vi "Teleop.vi"(10 "Match Info":T1={"Autonomous Elapsed Seconds"=0.0, "TeleOp Elapsed Seconds"=0.0, "Disabled Elapsed Seconds"=0.0, "Visited Autonomous"=FALSE, "Visited TeleOp"=FALSE, "Visited Disabled"=FALSE, "Autonomous Settings"={"Autonomous Style"=enum."Independent", "VI Refnum"=refnum}}, 11 "Call Context":T2) -> ()   [LabVIEW 2018]
doc: "This VI is called for each TeleOp packet received from the DS where the robot is not disabled. It is often used to read from the joysticks and update I/O or to update setpoints for timed control loops. It should complete and return within 20 milliseconds or it may miss DS packets."
uses:
  <vilib>/Rock Robotics/WPI/DriverStation/WPI_DriverStationDerivedRobotMode.ctl
  <vilib>/Rock Robotics/WPI/DriverStation/WPI_DriverStationMatch Info.ctl
  <vilib>/Rock Robotics/WPI/Utilities/WPI_GetSetVariantRefNum.vi
  <vilib>/Rock Robotics/Network Tables/NT Write Boolean Array.vi
  <vilib>/Rock Robotics/Network Tables/NT Write Numeric Array.vi
  <vilib>/Rock Robotics/Network Tables/NT Read Boolean.vi
  <vilib>/Rock Robotics/Network Tables/NT Read Number.vi
panel:
  out "Sample Slider 0":dbl(slide) scale=0.0..5.0
  out "Sample Boolean 1":bool
  out "Sample Boolean 0":bool
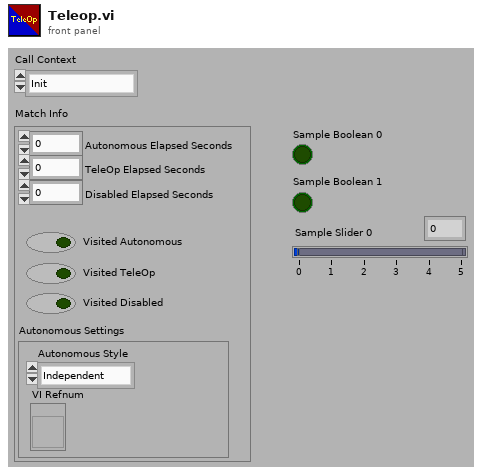
[diagram p1: front panel]
types:
  T1 = typedef "WPI_DriverStationMatch Info.ctl" = cluster{"Autonomous Elapsed Seconds":dbl, "TeleOp Elapsed Seconds":dbl, "Disabled Elapsed Seconds":dbl, "Visited Autonomous":bool, "Visited TeleOp":bool, "Visited Disabled":bool, "Autonomous Settings":cluster{"Autonomous Style":enum16{"Iterative", "Independent"}, "VI Refnum":refnum<vi>}}
  T2 = typedef "WPI_DriverStationDerivedRobotMode.ctl" = enum16{"Init", "Execute", "Stop"}
  T3 = typedef "WPI_RobotDriveDevRef.ctl" = cluster{"DevStatus":errorcluster, "Motors[]":T4[], "Square Inputs":bool, "Max Output":dbl}
  T4 = typedef "WPI_MotorControlDeviceRef.ctl" = cluster{"DeviceStatus":errorcluster, "Type":T5, "PWM":cluster{"PWM Channel":T6, "DeadBand":T7}, "CAN":cluster{"Device Number":u8, "SetOutput VI Ref":variant, "GetOutput VI Ref":variant, "Enable VI Ref":variant, "Disable VI Ref":variant, "Data":variant}, "Invert":bool, "DIO PWM":cluster{"PWM \"Enable\" Channel":T6, "DIOChannel":T8, "PWM Rate":dbl}}
  T5 = typedef "WPI_MotorControlType.ctl" = enum16{"PWM", "CAN", "DIO PWM"}
  T6 = typedef "FPGA_DIOPWMChannel.ctl" = enum8{"PWM 0", "PWM 1", "PWM 2", "PWM 3", "PWM 4", "PWM 5", "PWM 6", "PWM 7", "PWM 8", "PWM 9", "PWM MXP 0", "PWM MXP 1", "PWM MXP 2", "PWM MXP 3", "PWM MXP 4", "PWM MXP 5", "PWM MXP 6", "PWM MXP 7", "PWM MXP 8", "PWM MXP 9", "Invalid"}
  T7 = typedef "WPI_PWMDeadband.ctl" = cluster{"Name":string, "maxPositivePwm":i32, "minPositivePwm":i32, "centerPwm":i32, "maxNegativePwm":i32, "minNegativePwm":i32, "angularRange":u16}
  T8 = typedef "FPGA_DIOChannel.ctl" = enum8{"DIO 0", "DIO 1", "DIO 2", "DIO 3", "DIO 4", "DIO 5", "DIO 6", "DIO 7", "DIO 8", "DIO 9", "DIO MXP 0", "DIO MXP 1", "DIO MXP 2", "DIO MXP 3", "DIO MXP 4", "DIO MXP 5", "DIO MXP 6", "DIO MXP 7", "DIO MXP 8", "DIO MXP 9", "DIO MXP 10", "DIO MXP 11", "DIO MXP 12", "DIO MXP 13", "DIO MXP 14", "DIO MXP 15", "SPI Port CS1", "SPI Port CS2", "SPI Port CS3", "SPI Port MISO", "SPI Port MOSI", "Invalid"}
  T9 = typedef "WPI_JoystickDevRef.ctl" = cluster{"Device":T10}
  T10 = typedef "WPI_JoystickDeviceEnum.ctl" = enum16{"USB 0", "USB 1", "USB 2", "USB 3", "USB 4", "USB 5"}
  T11 = typedef "WPI_SwitchDevRef.ctl" = cluster{"DevStatus":errorcluster, "DIO Channel":T8, "CntIndex":T12, "Normally Closed":bool}
  T12 = typedef "FPGA_CounterCtrSystemIndex.ctl" = enum8{"Ctr 0", "Ctr 1", "Ctr 2", "Ctr 3", "Ctr 4", "Ctr 5", "Ctr 6", "Ctr 7", "Invalid"}
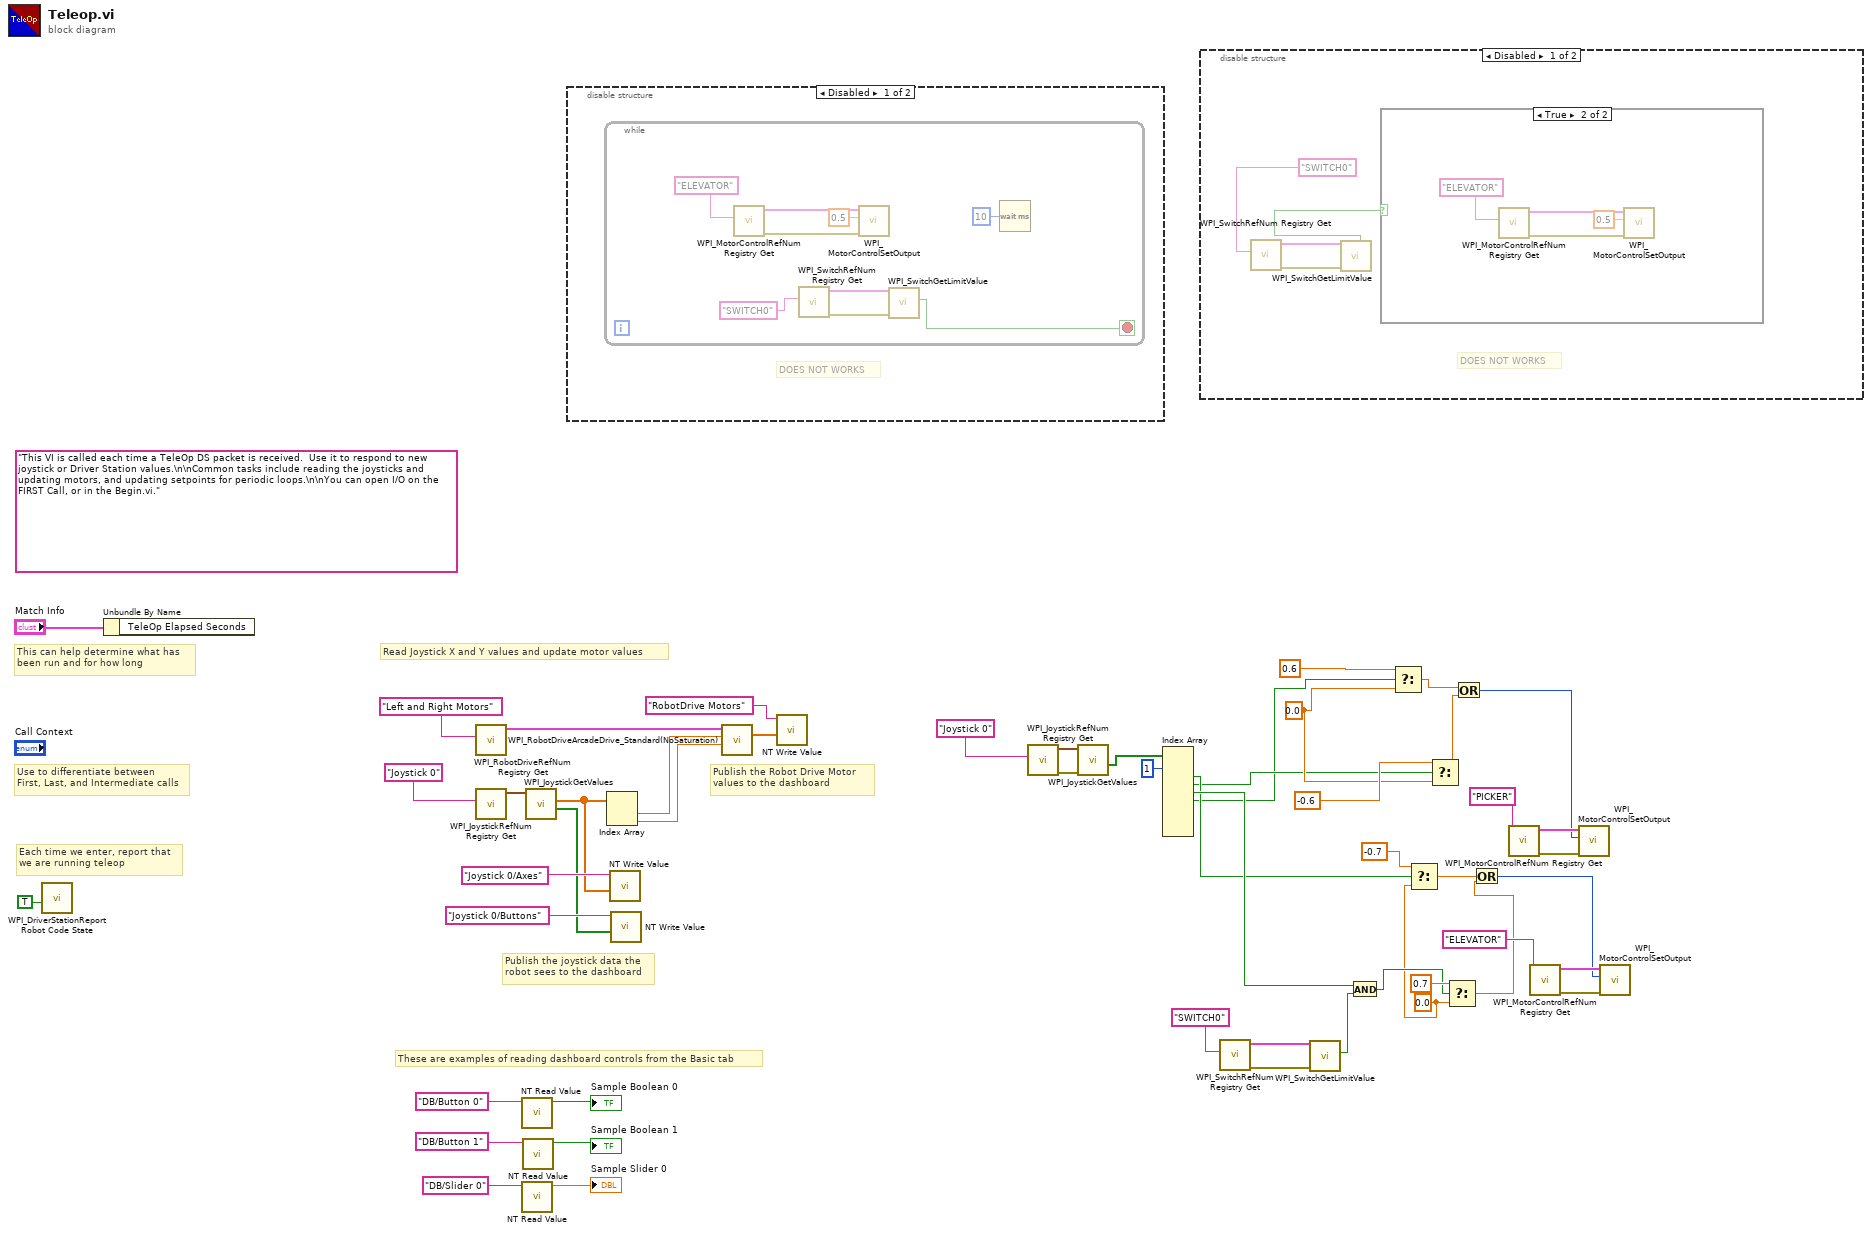
[diagram p0: block diagram]
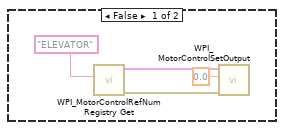
[diagram p2: hidden frame]
diagram:
  w4 = 0.0 ("f")
  w11 = 0.0 ("t")
  (unwired) "This VI is called each time a TeleOp DS packet is received.  Use it to respond to new joystick or Driver Station values.\n\nCommon tasks include reading the joysticks and updating motors, and updating setpoints for periodic loops.\n\nYou can open I/O on the FIRST Call, or in the Begin.vi."
  # "These are examples of reading dashboard controls from the Basic tab"
  # "Publish the Robot Drive Motor\nvalues to the dashboard"
  # "Publish the joystick data the\nrobot sees to the dashboard"
  # "Each time we enter, report that\nwe are running teleop"
  # "Use to differentiate between\nFirst, Last, and Intermediate calls"
  # "This can help determine what has\nbeen run and for how long"
  # "Read Joystick X and Y values and update motor values"
  n1 = call <vilib>:"WPI_DriverStationReport Robot Code State.vi"("TeleOp"=TRUE ("Autonomous")) -> ()  [unwired: 10 in, 1 out]
  n2 = Unbundle By Name("Match Info") -> ()  [unwired: 1 out]
  n3 = call <vilib>:"WPI_RobotDriveRefNum Registry Get.vi"("refnum name"="Left and Right Motors") -> ("RobotDriveDevRef"=w50:T3)  [unwired: 1 in, 9 out]
  n4 = call <vilib>:"WPI_JoystickRefNum Registry Get.vi"("refnum name"="Joystick 0") -> ("JoystickDevRef"=w47:T9)  [unwired: 1 in, 9 out]
  n5 = call-poly <vilib>:"NT Read Value.vi"("Name"="DB/Button 0" ("refnum name")) -> ("Boolean"=→"Sample Boolean 0":bool)  [unwired: 9 in, 1 out]
  n6 = call-poly <vilib>:"NT Read Value.vi"("Name"="DB/Slider 0" ("refnum name")) -> ("Numeric"=→"Sample Slider 0":dbl)  [unwired: 9 in, 1 out]
  n7 = call-poly <vilib>:"NT Read Value.vi"("Name"="DB/Button 1" ("refnum name")) -> ("Boolean"=→"Sample Boolean 1":bool)  [unwired: 9 in, 1 out]
  n8 = call <vilib>:"WPI_JoystickGetValues.vi"("JoystickDevRef"=w47) -> ("Buttons"=w41:bool[], "Axes"=w42:dbl[])  [unwired: 6 in, 3 out]
  n9 = disable-structure shown="Disabled" {
    frame Disabled {
      # "DOES NOT WORKS"
      n10 = while {
        stop <- w53 stop-if-true
        n11 = call <vilib>:"WPI_MotorControlRefNum Registry Get.vi"("refnum name"="ELEVATOR") -> ("error out"=w58:errorcluster, "MotorControlDevRef"=w57:T4)  [unwired: 9 in]
        n12 = call <vilib>:"WPI_SwitchRefNum Registry Get.vi"("refnum name"="SWITCH0") -> ("error out"=w61:errorcluster, "SwitchDevRef"=w60:T11)  [unwired: 9 in]
        n13 = call <vilib>:"WPI_MotorControlSetOutput.vi"("error in (no error)"=w58, "Output"=0.5, "MotorControlDevRef"=w57) -> ()  [unwired: 6 in, 3 out]
        n14 = call <vilib>:"WPI_SwitchGetLimitValue.vi"("error in (no error)"=w61, "SwitchDevRef"=w60) -> ("Switch Pressed"=w53:bool)  [unwired: 7 in, 2 out]
        n15 = Wait (ms)(milliseconds to wait=u32 10) -> ()  [unwired: 1 out]
      }
    }
    frame Enabled {
    }
  }
  n16 = Index Array(array=w42) -> (element #1=w49:dbl, element #2=w45:dbl)  [unwired: 2 in]
  n17 = call-poly <vilib>:"NT Write Value.vi"("Numeric Array"=w42, "Name"="Joystick 0/Axes") -> ()  [unwired: 9 in, 1 out]
  n18 = call-poly <vilib>:"NT Write Value.vi"("Boolean Array"=w41, "Name"="Joystick 0/Buttons") -> ()  [unwired: 9 in, 1 out]
  n19 = call <vilib>:"WPI_RobotDriveArcadeDrive_Standard(NoSaturation).vi"("Y axis value"=w45, "X axis value"=w49, "RobotDriveDevRef"=w50) -> ("Motor Values"=w34:dbl[])  [unwired: 1 in, 7 out]
  n20 = call-poly <vilib>:"NT Write Value.vi"("Numeric Array"=w34, "Name"="RobotDrive Motors") -> ()  [unwired: 9 in, 1 out]
  n21 = call <vilib>:"WPI_JoystickRefNum Registry Get.vi"("refnum name"="Joystick 0") -> ("error out"=w28:errorcluster, "JoystickDevRef"=w31:T9)  [unwired: 1 in, 8 out]
  n22 = call <vilib>:"WPI_JoystickGetValues.vi"("error in (no error)"=w28, "JoystickDevRef"=w31) -> ("Buttons"=w30:bool[])  [unwired: 5 in, 4 out]
  n23 = Index Array(array=w30, index #1=1 ("index")) -> (element #2=w3:bool, element #3=w2:bool, element #4=w9:bool, element #5=w1:bool)  [unwired: 8 in, 5 out]
  n24 = disable-structure shown="Disabled" {
    frame Disabled {
      # "DOES NOT WORKS"
      n25 = call <vilib>:"WPI_SwitchRefNum Registry Get.vi"("refnum name"="SWITCH0") -> ("error out"=w65:errorcluster, "SwitchDevRef"=w64:T11)  [unwired: 9 in]
      n26 = call <vilib>:"WPI_SwitchGetLimitValue.vi"("error in (no error)"=w65, "SwitchDevRef"=w64) -> ("Switch Pressed"=w62:bool)  [unwired: 7 in, 2 out]
      n27 = case shown="True" w62 {
        frame False {
          n28 = call <vilib>:"WPI_MotorControlRefNum Registry Get.vi"("refnum name"="ELEVATOR") -> ("error out"=w69:errorcluster, "MotorControlDevRef"=w68:T4)  [unwired: 9 in]
          n29 = call <vilib>:"WPI_MotorControlSetOutput.vi"("error in (no error)"=w69, "Output"=0.0, "MotorControlDevRef"=w68) -> ()  [unwired: 6 in, 3 out]
        }
        frame True {
          n30 = call <vilib>:"WPI_MotorControlRefNum Registry Get.vi"("refnum name"="ELEVATOR") -> ("error out"=w73:errorcluster, "MotorControlDevRef"=w72:T4)  [unwired: 9 in]
          n31 = call <vilib>:"WPI_MotorControlSetOutput.vi"("error in (no error)"=w73, "Output"=0.5, "MotorControlDevRef"=w72) -> ()  [unwired: 6 in, 3 out]
        }
      }
    }
    frame Enabled {
    }
  }
  n32 = call <vilib>:"WPI_SwitchRefNum Registry Get.vi"("refnum name"="SWITCH0") -> ("error out"=w17:errorcluster, "SwitchDevRef"=w19:T11)  [unwired: 9 in]
  n33 = call <vilib>:"WPI_SwitchGetLimitValue.vi"("error in (no error)"=w17, "SwitchDevRef"=w19) -> ("Switch Pressed"=w15:bool)  [unwired: 7 in, 2 out]
  n34 = And(x=w9, y=w15) -> (x .and. y?=w16:bool)
  n35 = Select(t=0.6, s=w1, f=w11) -> (s? t:f=w14:dbl)
  n36 = Select(t=-0.7, s=w3, f=w4) -> (s? t:f=w7:dbl)
  n37 = Select(t=-0.6, s=w2, f=w11) -> (s? t:f=w10:dbl)
  n38 = Select(t=0.7, s=w16, f=w4) -> (s? t:f=w8:dbl)
  n39 = Or(x=w14, y=w10) -> (x .or. y?=w13:i32)
  n40 = Or(x=w7, y=w8) -> (x .or. y?=w6:i32)
  n41 = call <vilib>:"WPI_MotorControlRefNum Registry Get.vi"("refnum name"="PICKER") -> ("error out"=w25:errorcluster, "MotorControlDevRef"=w26:T4)  [unwired: 9 in]
  n42 = call <vilib>:"WPI_MotorControlRefNum Registry Get.vi"("refnum name"="ELEVATOR") -> ("error out"=w21:errorcluster, "MotorControlDevRef"=w22:T4)  [unwired: 9 in]
  n43 = call <vilib>:"WPI_MotorControlSetOutput.vi"("error in (no error)"=w25, "Output"=w13, "MotorControlDevRef"=w26) -> ()  [unwired: 6 in, 3 out]
  n44 = call <vilib>:"WPI_MotorControlSetOutput.vi"("error in (no error)"=w21, "Output"=w6, "MotorControlDevRef"=w22) -> ()  [unwired: 6 in, 3 out]
